vi "testVariants.vi"() -> ()   [LabVIEW 2013]
panel:
  out "variant out":variant
  out "ageOut":dbl
  out "error out 2":errorcluster
  out "error out":errorcluster
  in  "ageIn":dbl
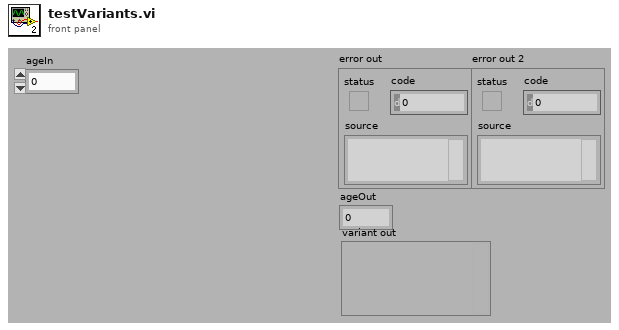
[diagram p1: front panel]
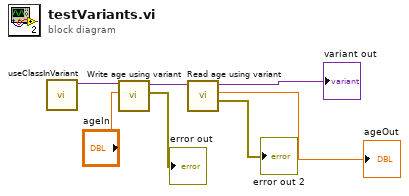
[diagram p0: block diagram]
diagram:
  n1 = call "useClassInVariant.vi"() -> ("variant"=w7:variant)  [unwired: 11 in]
  n2 = call "Write age using variant.vi"("age"="ageIn", "variant in"=w7) -> ("error out"=→"error out":errorcluster, "variant out"=w6:variant)  [unwired: 8 in]
  n3 = call "Read age using variant.vi"("variant in"=w6) -> ("error out"=→"error out 2":errorcluster, "age"=→"ageOut":dbl, "variant out"=→"variant out":variant)  [unwired: 8 in]
